vi "Wait (SubVI).vi"(10 "Wait? (T)":bool=TRUE, 11 "Occurrence in":refnum<k4>) -> ()   [LabVIEW 2017]
uses:
  <vilib>/rvi/occurrence/nirviWaitOnOccurrenceBase.vi
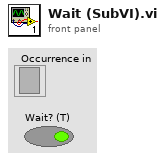
[diagram p1: front panel]
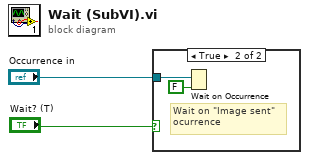
[diagram p0: block diagram]
diagram:
  n1 = case shown="True" "Wait? (T)" {
    tunnel: "Occurrence in" -> [_ w4]
    frame False {
    }
    frame True {
      # "Wait on \"Image sent\"\nocurrence"
      n2 = Wait on Occurrence(1:FALSE ("ignore previous (T)"), 2:w4) -> ()  [unwired: 1 in, 1 out]
    }
  }
